vi "Do Request.vi"(7 "Processing In":refnum<class "Processing.lvclass">, 11 "SequencingHttpCtrlr in":refnum<class "SequencingHttpCtrlr.lvclass">) -> (0 "error out":errorcluster, 5 "Processing":refnum<class "Processing.lvclass">)   [LabVIEW 2020, in "VolatusSeq.lvlib" / "SequencingHttpCtrlr.lvclass"]
doc: "A controller's main job is to respond to a request by generating a response. The response value must be specified by calling Set Response.vi on the Processing class that's passed through the VI otherwise an error will be generated.\n\nThere are several helpers available for common response types:\nGenerating HTML content programmatically - Create Basic Response.vi\nStreaming a file from disk - Create File Response.vi\nRedirecting the user to another URL - Create Redirect Response.vi\n\nFile responses are streamed in chunks and do not load the entire file into memory at once to send in the response which allows serving large files more efficiently."
uses:
  SequencingHttpCtrlr.lvclass
  lv-http-server/HTTP Server/Processing/Processing.lvclass
  SequencingHttpCtrlr.lvclass/SequencingHttpCtrlr.ctl
  lv-http-server/HTTP Server/Processing/Processing.lvclass/Processing.ctl
  lv-http-util/HTTP Utils/Request/Request.lvclass/Request.ctl
  lv-uri/URI/URI/URI.lvclass/URI.ctl
  Sequence Load Data.ctl
  lv-promises/Promises/Value/Value.lvclass
  Sequencing Status Value/Sequencing Status Value.lvclass
  Sequencing Status Value/Sequencing Status Value.lvclass/Sequencing Status Value.ctl
  lv-http-util/HTTP Utils/Request/Get Target URI.vi
  lv-uri/URI/URI/Path String.vi
  Sequencing Status Value/Read.vi
  lv-vecto/Vecto/Double Timestamp to Unix ns.vi
  lv-vecto/Vecto/Double to Relative ns.vi
  lv-http-util/HTTP Utils/Request/Request.lvclass
  lv-http-util/HTTP Utils/FormField/FormField.lvclass
  VolatusSeq.lvlib
  Volatus/MessageQ/MessageQ.lvclass
  lv-http-util/HTTP Utils/Response/Response.lvclass
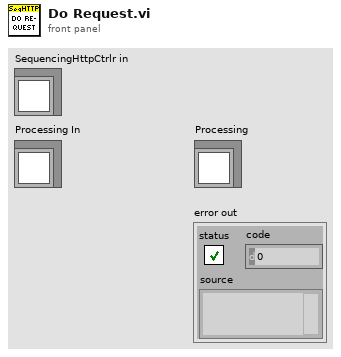
[diagram p1: front panel]
types:
  T1 = typedef "VolatusSeq.lvlib/Sequence Load Data.ctl" = cluster{"Name":string, "JSON":string, "Hash":string}
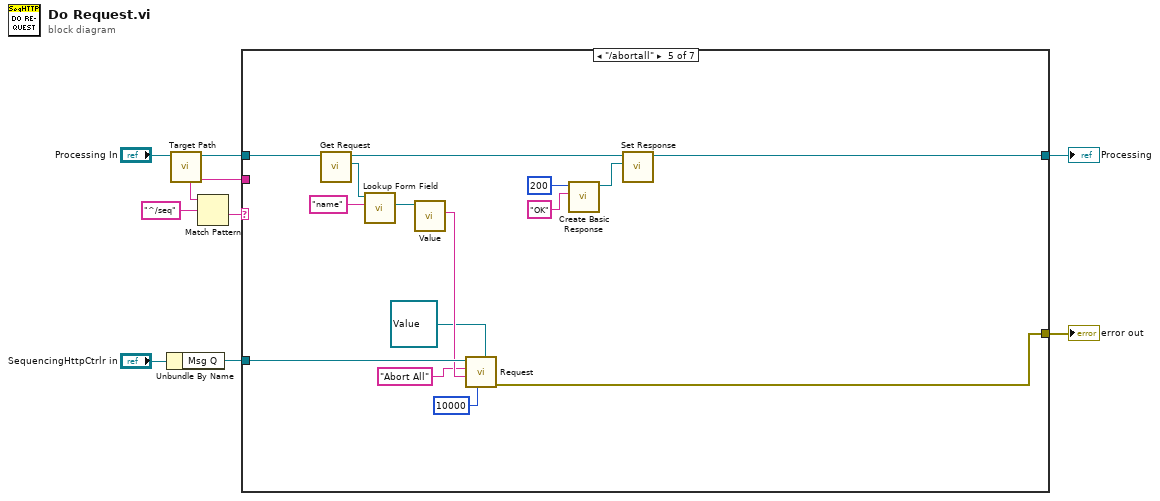
[diagram p0: block diagram]
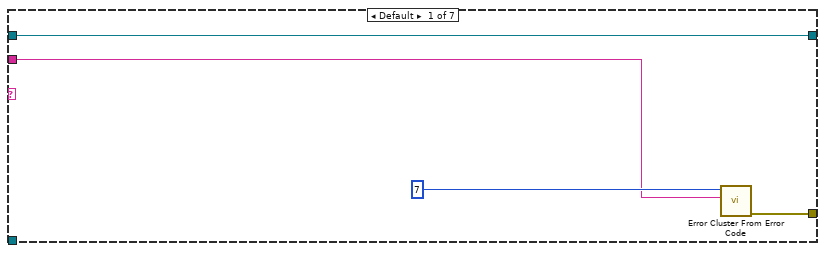
[diagram p2: hidden frame]
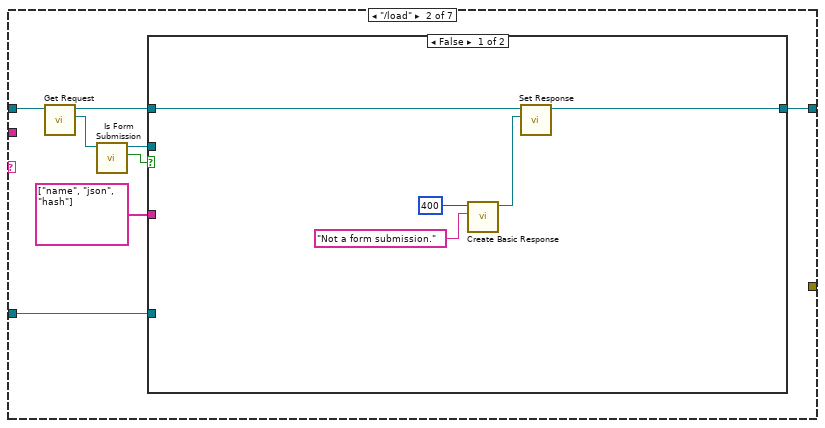
[diagram p3: hidden frame]
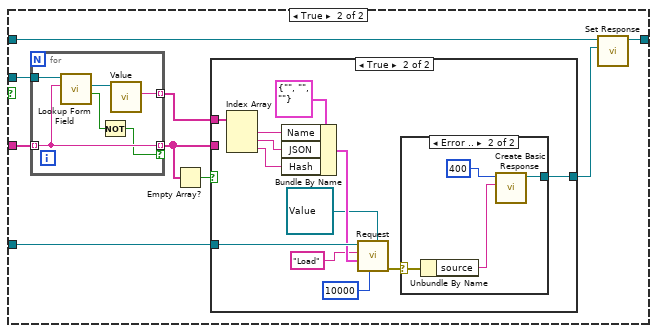
[diagram p4: hidden frame]
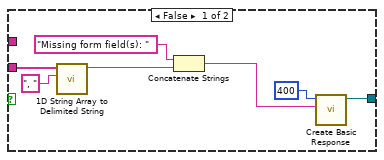
[diagram p5: hidden frame]
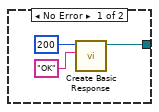
[diagram p6: hidden frame]
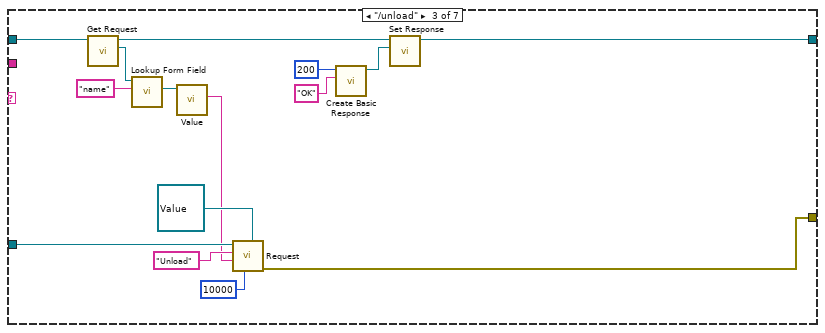
[diagram p7: hidden frame]
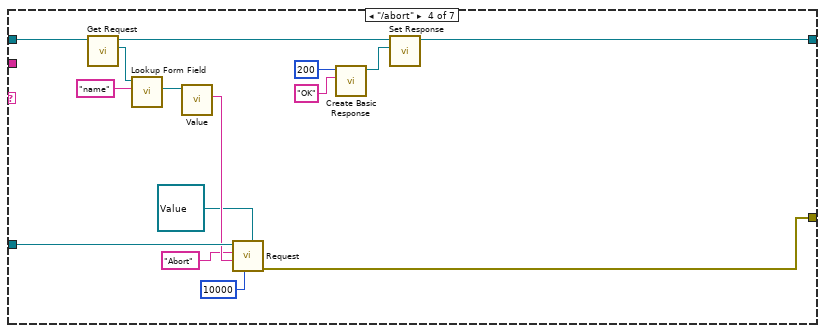
[diagram p8: hidden frame]
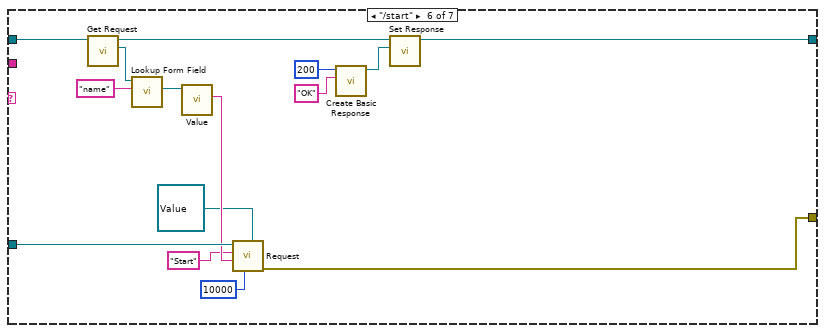
[diagram p9: hidden frame]
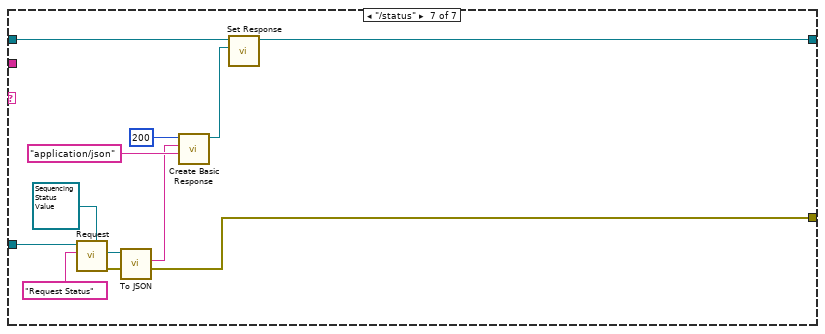
[diagram p10: hidden frame]
diagram:
  n1 = Unbundle By Name("SequencingHttpCtrlr in") -> ("Msg Q"=w4:refnum<class "MessageQ.lvclass">)
  n2 = call "Target Path.vi"("Processing in"="Processing In") -> ("Processing out"=w5:refnum<class "Processing.lvclass">, "Target Path"=w3:string)  [unwired: 9 in]
  n3 = Match Pattern(string=w3, regular expression="^/seq") -> (after substring=w6:string)  [unwired: 1 in, 3 out]
  n4 = case shown="\"/abortall\"" w6 {
    tunnel: w5 -> [w10 w21 w82 w97 w112 w127 w131]
    tunnel: w4 -> [_ w15 w79 w93 w108 w123 w138]
    tunnel: w3 -> [w12 _ _ _ _ _ _]
    tunnel: [w11 _ w76 w89 w104 w119 w128] -> w2
    tunnel: [w10 w14 w70 w83 w98 w113 w129] -> w1
    frame Default {
      n5 = call <vilib>:"Error Cluster From Error Code.vi"("error message (\"\")"=w12, "error code (0)"=7) -> ("error out"=w11:errorcluster)  [unwired: 7 in]
    }
    frame "/load" {
      n6 = call "Get Request.vi"("Processing in"=w21) -> ("Request"=w20:refnum<class "Request.lvclass">, "Processing out"=w19:refnum<class "Processing.lvclass">)  [unwired: 9 in]
      n7 = call "Is Form Submission.vi"("Request in"=w20) -> ("Is Form Submission?"=w17:bool, "Request out"=w18:refnum<class "Request.lvclass">)  [unwired: 8 in, 1 out]
      n8 = case shown="False" w17 {
        tunnel: w19 -> [w26 w31]
        tunnel: w18 -> [_ w35]
        tunnel: string[] ["name", "json", "hash"] -> [_ w34]
        tunnel: w15 -> [_ w32]
        tunnel: [w23 w30] -> w14
        frame False {
          n9 = call "Create Basic Response.vi"("Payload"="Not a form submission." ("error message (\"\")"), "Status Code"=u16 400) -> ("Response out"=w22:refnum<class "Response.lvclass">)  [unwired: 8 in, 1 out]
          n10 = call "Set Response.vi"("Response"=w22, "Processing in"=w26) -> ("Processing out"=w23:refnum<class "Processing.lvclass">)  [unwired: 9 in]
        }
        frame True {
          n11 = for {
            tunnel: w35 -> [w67]
            tunnel: w34 -> [w66] mode=indexing
            tunnel: [w66] -> w28 mode=indexing if=w64
            tunnel: [w62] -> w33 mode=indexing
            n12 = call "Lookup Form Field.vi"("Name"=w66, "Request in"=w67) -> ("Exists"=w65:bool, "Field"=w63:refnum<class "FormField.lvclass">)  [unwired: 6 in, 2 out]
            n13 = Not(x=w65) -> (.not. x?=w64:bool)
            n14 = call "Value.vi"("FormField in"=w63) -> ("Value"=w62:string)  [unwired: 8 in, 2 out]
          }
          n15 = Empty Array?(array=w28) -> (empty?=w29:bool)
          n16 = case shown="True" w29 {
            tunnel: w33 -> [_ w54]
            tunnel: w32 -> [_ w49]
            tunnel: w28 -> [w42 _]
            tunnel: [w38 w43] -> w27
            frame False {
              n17 = call <vilib>:"1D String Array to Delimited String.vi"("delimiter"=", ", "string array"=w42) -> ("delimited string"=w40:string)  [unwired: 9 in]
              n18 = Concatenate Strings("Missing form field(s): ", w40) -> (w36:string)
              n19 = call "Create Basic Response.vi"("Payload"=w36, "Status Code"=u16 400) -> ("Response out"=w38:refnum<class "Response.lvclass">)  [unwired: 8 in, 1 out]
            }
            frame True {
              n20 = Index Array(array=w54) -> (element #1=w52:string, element #2=w51:string, element #3=w50:string)  [unwired: 3 in]
              n21 = Bundle By Name(cluster=T1 {"Name"="", "JSON"="", "Hash"=""} ("Sequence Load Data"), "Name"=w52, "JSON"=w51, "Hash"=w50) -> (w48:T1)
              n22 = call "Request.vi"("Response Type (None)"=refnum<class "Value.lvclass"> refnum ("Response Value Type"), "Timeout ms (1000)"=10000, "Data"=w48, "ID"="Load", "MessageQ in"=w49) -> ("error out"=w44:errorcluster)  [unwired: 4 in, 2 out]
              n23 = case shown="Error .." w44 {
                selector: w44 -> [_ w59]
                tunnel: [w55 w61] -> w43
                frame No Error {
                  n24 = call "Create Basic Response.vi"("Payload"="OK", "Status Code"=u16 200) -> ("Response out"=w55:refnum<class "Response.lvclass">)  [unwired: 8 in, 1 out]
                }
                frame Error {
                  n25 = Unbundle By Name(w59) -> ("source"=w58:string)
                  n26 = call "Create Basic Response.vi"("Payload"=w58, "Status Code"=u16 400) -> ("Response out"=w61:refnum<class "Response.lvclass">)  [unwired: 8 in, 1 out]
                }
              }
            }
          }
          n27 = call "Set Response.vi"("Response"=w27, "Processing in"=w31) -> ("Processing out"=w30:refnum<class "Processing.lvclass">)  [unwired: 9 in]
        }
      }
    }
    frame "/unload" {
      n28 = call "Get Request.vi"("Processing in"=w82) -> ("Request"=w81:refnum<class "Request.lvclass">, "Processing out"=w72:refnum<class "Processing.lvclass">)  [unwired: 9 in]
      n29 = call "Lookup Form Field.vi"("Name"="name", "Request in"=w81) -> ("Field"=w69:refnum<class "FormField.lvclass">)  [unwired: 6 in, 3 out]
      n30 = call "Value.vi"("FormField in"=w69) -> ("Value"=w68:string)  [unwired: 8 in, 2 out]
      n31 = call "Request.vi"("Response Type (None)"=refnum<class "Value.lvclass"> refnum ("Response Value Type"), "Timeout ms (1000)"=10000, "Data"=w68, "ID"="Unload", "MessageQ in"=w79) -> ("error out"=w76:errorcluster)  [unwired: 4 in, 2 out]
      n32 = call "Create Basic Response.vi"("Payload"="OK", "Status Code"=u16 200) -> ("Response out"=w71:refnum<class "Response.lvclass">)  [unwired: 8 in, 1 out]
      n33 = call "Set Response.vi"("Response"=w71, "Processing in"=w72) -> ("Processing out"=w70:refnum<class "Processing.lvclass">)  [unwired: 9 in]
    }
    frame "/abort" {
      n34 = call "Get Request.vi"("Processing in"=w97) -> ("Request"=w96:refnum<class "Request.lvclass">, "Processing out"=w85:refnum<class "Processing.lvclass">)  [unwired: 9 in]
      n35 = call "Lookup Form Field.vi"("Name"="name", "Request in"=w96) -> ("Field"=w94:refnum<class "FormField.lvclass">)  [unwired: 6 in, 3 out]
      n36 = call "Value.vi"("FormField in"=w94) -> ("Value"=w92:string)  [unwired: 8 in, 2 out]
      n37 = call "Request.vi"("Response Type (None)"=refnum<class "Value.lvclass"> refnum ("Response Value Type"), "Timeout ms (1000)"=10000, "Data"=w92, "ID"="Abort", "MessageQ in"=w93) -> ("error out"=w89:errorcluster)  [unwired: 4 in, 2 out]
      n38 = call "Create Basic Response.vi"("Payload"="OK", "Status Code"=u16 200) -> ("Response out"=w84:refnum<class "Response.lvclass">)  [unwired: 8 in, 1 out]
      n39 = call "Set Response.vi"("Response"=w84, "Processing in"=w85) -> ("Processing out"=w83:refnum<class "Processing.lvclass">)  [unwired: 9 in]
    }
    frame "/abortall" {
      n40 = call "Get Request.vi"("Processing in"=w112) -> ("Request"=w111:refnum<class "Request.lvclass">, "Processing out"=w100:refnum<class "Processing.lvclass">)  [unwired: 9 in]
      n41 = call "Lookup Form Field.vi"("Name"="name", "Request in"=w111) -> ("Field"=w109:refnum<class "FormField.lvclass">)  [unwired: 6 in, 3 out]
      n42 = call "Value.vi"("FormField in"=w109) -> ("Value"=w107:string)  [unwired: 8 in, 2 out]
      n43 = call "Request.vi"("Response Type (None)"=refnum<class "Value.lvclass"> refnum ("Response Value Type"), "Timeout ms (1000)"=10000, "Data"=w107, "ID"="Abort All", "MessageQ in"=w108) -> ("error out"=w104:errorcluster)  [unwired: 4 in, 2 out]
      n44 = call "Create Basic Response.vi"("Payload"="OK", "Status Code"=u16 200) -> ("Response out"=w99:refnum<class "Response.lvclass">)  [unwired: 8 in, 1 out]
      n45 = call "Set Response.vi"("Response"=w99, "Processing in"=w100) -> ("Processing out"=w98:refnum<class "Processing.lvclass">)  [unwired: 9 in]
    }
    frame "/start" {
      n46 = call "Get Request.vi"("Processing in"=w127) -> ("Request"=w126:refnum<class "Request.lvclass">, "Processing out"=w115:refnum<class "Processing.lvclass">)  [unwired: 9 in]
      n47 = call "Lookup Form Field.vi"("Name"="name", "Request in"=w126) -> ("Field"=w124:refnum<class "FormField.lvclass">)  [unwired: 6 in, 3 out]
      n48 = call "Value.vi"("FormField in"=w124) -> ("Value"=w122:string)  [unwired: 8 in, 2 out]
      n49 = call "Request.vi"("Response Type (None)"=refnum<class "Value.lvclass"> refnum ("Response Value Type"), "Timeout ms (1000)"=10000, "Data"=w122, "ID"="Start", "MessageQ in"=w123) -> ("error out"=w119:errorcluster)  [unwired: 4 in, 2 out]
      n50 = call "Create Basic Response.vi"("Payload"="OK", "Status Code"=u16 200) -> ("Response out"=w114:refnum<class "Response.lvclass">)  [unwired: 8 in, 1 out]
      n51 = call "Set Response.vi"("Response"=w114, "Processing in"=w115) -> ("Processing out"=w113:refnum<class "Processing.lvclass">)  [unwired: 9 in]
    }
    frame "/status" {
      n52 = call "Request.vi"("Response Type (None)"=refnum<class "Sequencing Status Value.lvclass"> refnum ("VolatusSeq.lvlib:Sequencing Status Value.lvclass"), "ID"="Request Status", "MessageQ in"=w138) -> ("error out"=w128:errorcluster, "Response"=w135:refnum<class "Sequencing Status Value.lvclass">)  [unwired: 6 in, 1 out]
      n53 = call "To JSON.vi"("Sequencing Status Value in"=w135) -> ("Status JSON"=w133:string)  [unwired: 10 in]
      n54 = call "Create Basic Response.vi"("Content-Type (text/plain)"="application/json", "Payload"=w133, "Status Code"=u16 200) -> ("Response out"=w130:refnum<class "Response.lvclass">)  [unwired: 7 in, 1 out]
      n55 = call "Set Response.vi"("Response"=w130, "Processing in"=w131) -> ("Processing out"=w129:refnum<class "Processing.lvclass">)  [unwired: 9 in]
    }
  }
  "error out" <- w2
  "Processing" <- w1
